vi "recording.vi"(6 "Data":dbl[](array[numeric]), 7 "Data 2":dbl[](array[numeric]), 9 "Queue in":refnum<queue>, 10 "recording":bool, 11 "cluster in in":T1) -> (3 "cluster out":T1)   [LabVIEW 2016]
doc: "update recording data if recrord is true, and check if 2 seconds have passed since start of record.\nif true, send stopWeak command"
uses:
  DataType.ctl
  data_command_enum.ctl
  DataLoopCluster.ctl
  SignalType.ctl
  range_cluster.ctl
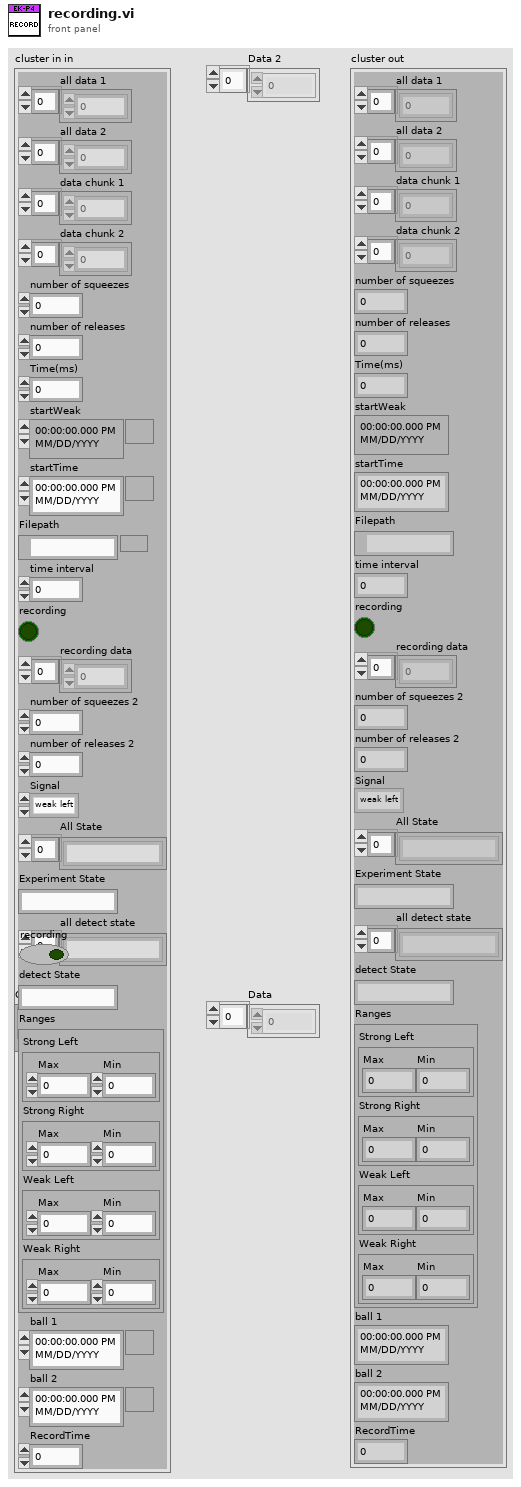
[diagram p1: front panel]
types:
  T1 = typedef "DataLoopCluster.ctl" = cluster{"all data 1":dbl[], "all data 2":dbl[], "data chunk 1":dbl[], "data chunk 2":dbl[], "number of squeezes":u16, "number of releases":u16, "Time(ms)":i64, "startWeak":timestamp, "startTime":timestamp, "Filepath":path, "time interval":u16, "recording":bool, "recording data":dbl[], "number of squeezes 2":u16, "number of releases 2":u16, "Signal":T2, "All State":string[], "Experiment State":string, "all detect state":string[], "detect State":string, "Ranges":cluster{"Strong Left":T3, "Strong Right":T3, "Weak Left":T3, "Weak Right":T3}, "ball 1":timestamp, "ball 2":timestamp, "RecordTime":u16}
  T2 = typedef "SignalType.ctl" = enum16{"weak left", "weak right", "strong left", "strong right"}
  T3 = typedef "range_cluster.ctl" = cluster{"Max":dbl, "Min":dbl}
  T4 = typedef "DataType.ctl" = cluster{"command":T5, "data":variant}
  T5 = typedef "data_command_enum.ctl" = enum16{"data", "display", "quit", "save", "filepath", "weak left", "state", "weak right", "strong left", "strong right", "stopRecording", "close", "sid"}
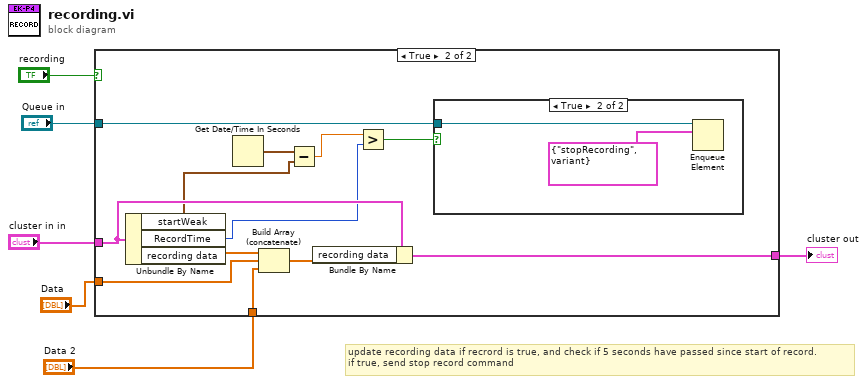
[diagram p0: block diagram]
diagram:
  # "update recording data if recrord is true, and check if 5 seconds have passed since start of record.\nif true, send stop record command"
  n1 = case shown="True" "recording" {
    tunnel: "Data" -> [_ w10]
    tunnel: "cluster in in" -> [w7 w19]
    tunnel: [w7 w18] -> w5
    tunnel: "Queue in" -> [_ w14]
    tunnel: "Data 2" -> [_ w9]
    frame False {
    }
    frame True {
      n2 = Unbundle By Name(w19) -> ("startWeak"=w11:timestamp, "RecordTime"=w8:u16, "recording data"=w12:dbl[])
      n3 = Get Date/Time In Seconds() -> (seconds since 1Jan1904=w16:timestamp)
      n4 = Build Array (concatenate)(w12, w10, w9) -> (w17:dbl[])
      n5 = Subtract(x=w16, y=w11) -> (x-y=w15:dbl)
      n6 = Bundle By Name(cluster=w19, "recording data"=w17) -> (w18:T1)
      n7 = Greater?(x=w15, y=w8) -> (0:w13:bool)
      n8 = case shown="True" w13 {
        tunnel: w14 -> [_ w21]
        frame False {
        }
        frame True {
          n9 = Enqueue Element(queue=w21, element=T4 {"command"=enum."stopRecording", "data"=variant}) -> ()  [unwired: 2 in, 3 out]
        }
      }
    }
  }
  "cluster out" <- w5
